vi "Synthesize.vi"(0 "FM Sweep in":refnum<class "FM Sweep.lvclass">, 5 "Fs (Hz)":dbl, 7 "Npts":i32, 9 "Repetition":i32, 11 "error in (no error)":errorcluster) -> (4 "FM Sweep out":refnum<class "FM Sweep.lvclass">, 8 "Array":dbl[](array[numeric]), 15 "error out":errorcluster)   [LabVIEW 2020, in "FM Sweep.lvclass"]
uses:
  FM Sweep.lvclass
  FM Sweep.lvclass/FM Sweep.ctl
  9b3f6198-7ac8-4a58-a697-dace7bb9d9f3.vi
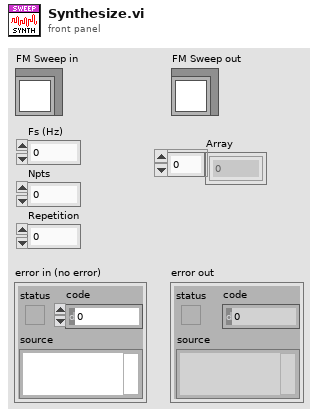
[diagram p1: front panel]
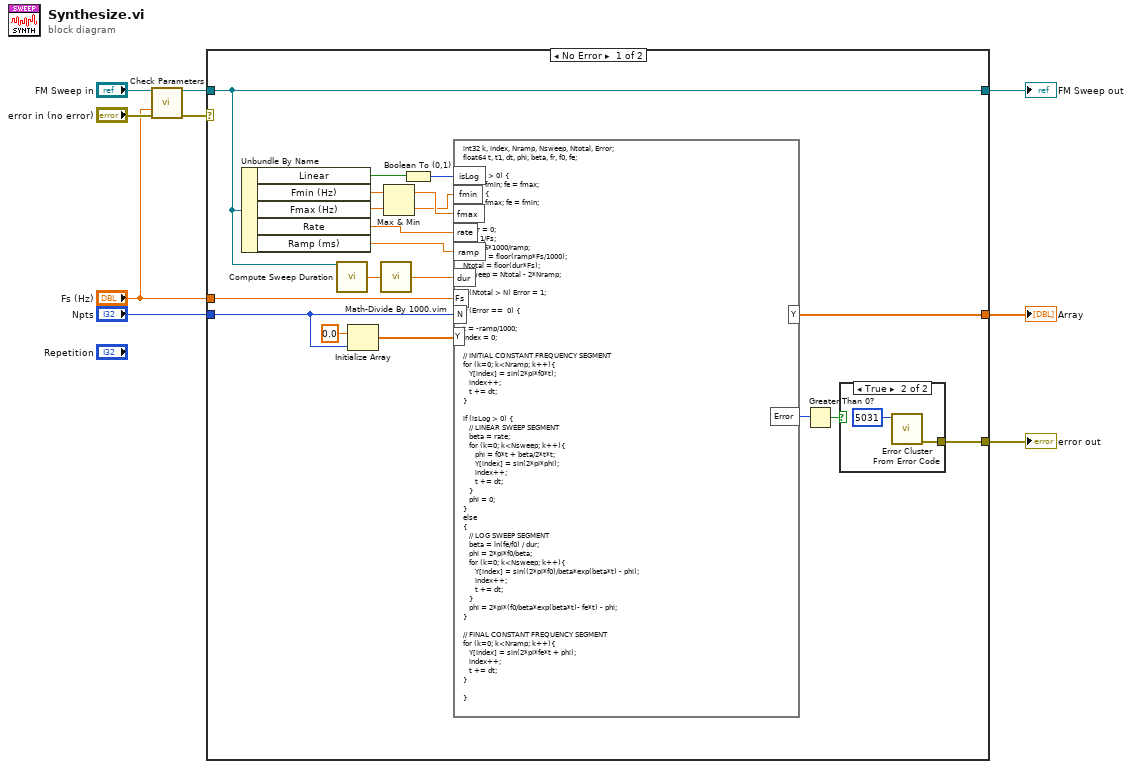
[diagram p0: block diagram]
diagram:
  n1 = call "Check Parameters.vi"("FM Sweep in"="FM Sweep in", "Fs (Hz)"="Fs (Hz)", "error in (no error)"="error in (no error)") -> ("FM Sweep out"=w5:refnum<class "FM Sweep.lvclass">, "error out"=w3:errorcluster)  [unwired: 11 in]
  n2 = case shown="No Error" w3 {
    selector: w3 -> [_ w31]
    tunnel: [w22 w31] -> w2
    tunnel: [w20 w32] -> w9
    tunnel: w5 -> [w20 w32]
    tunnel: "Npts" -> [w25 _]
    tunnel: "Fs (Hz)" -> [w27 _]
    tunnel: [w26 _] -> w7
    frame No Error {
      n3 = Unbundle By Name(w20) -> ("Linear"=w15:bool, "Fmin (Hz)"=w13:dbl, "Fmax (Hz)"=w12:dbl, "Rate"=w28:dbl, "Ramp (ms)"=w21:dbl)
      n4 = call "Compute Sweep Duration.vi"("FM Sweep in"=w20) -> ("Duration (ms)"=w19:dbl)  [unwired: 12 in, 2 out]
      n5 = Initialize Array(0.0 ("element"), w25) -> (w23:dbl[])
      n6 = call "Math-Divide By 1000.vim"("X"=w19) -> ("1000X"=w18:dbl)
      n7 = Max & Min(x=w13, y=w12) -> (max(x,y)=w11:dbl, min(x,y)=w10:dbl)
      n8 = Boolean To (0,1)(Boolean=w15) -> (0, 1=w14:i16)
      n9 = formula code="int32 k, index, Nramp, Nsweep, Ntotal, Error;\nfloat64 t, t1, dt, phi, beta, fr, f0, fe;\n\nif (rate > 0) {\n   f0 = fmin; fe = fmax;\n} else {\n   f0 = fmax; fe = fmin;\n}\n\nError = 0;\ndt = 1/Fs;\nfr = 0.5*1000/ramp;\nNramp = floor(ramp*Fs/1000);\nNtotal = floor(dur*Fs);\nNsweep = Ntotal - 2*Nramp;\n\nif (Ntotal > N) Error = 1;  \n\nif (Error ==  0) {\n\nt = -ramp/1000;\nindex = 0;\n\n// INITIAL CONSTANT FREQUENCY SEGMENT\nfor (k=0; k<Nramp; k++){\n   Y[index] = sin(2*pi*f0*t);  \n   index++;\n   t += dt;\n}\n\nif (isLog > 0) {\n   // LINEAR SWEEP SEGMENT\n   beta = rate;\n   for (k=0; k<Nsweep; k++){\n      phi = f0*t + beta/2*t*t;\n      Y[index] = sin(2*pi*phi);\n      index++;\n      t += dt;\n   }\n   phi = 0;\n}\nelse\n{\n   // LOG SWEEP SEGMENT\n   beta = ln(fe/f0) / dur;\n   phi = 2*pi*f0/beta;\n   for (k=0; k<Nsweep; k++){\n      Y[index] = sin((2*pi*f0)/beta*exp(beta*t) - phi);\n      index++;\n      t += dt;\n   }\n   phi = 2*pi*(f0/beta*exp(beta*t)- fe*t) - phi;\n}\n\n// FINAL CONSTANT FREQUENCY SEGMENT\nfor (k=0; k<Nramp; k++){\n   Y[index] = sin(2*pi*fe*t + phi);\n   index++;\n   t += dt;\n}\n\n}"("fmin"=w10, "fmax"=w11, "rate"=w28, "ramp"=w21, "Fs"=w27, "N"=w25, "Y"=w23, "dur"=w18, "isLog"=w14) -> ("Y"=w26:dbl[], "Error"=w17:i32)
      n10 = Greater Than 0?(x=w17) -> (x > 0?=w16:bool)
      n11 = case shown="True" w16 {
        tunnel: [_ w29] -> w22
        frame False {
        }
        frame True {
          n12 = call <vilib>:"Error Cluster From Error Code.vi"("error code (0)"=5031) -> ("error out"=w29:errorcluster)  [unwired: 8 in]
        }
      }
    }
    frame Error {
    }
  }
  "error out" <- w2
  "FM Sweep out" <- w9
  "Array" <- w7
